vi "Test Person Updates Status on Trigger Broadcast.vi"(8 "error in (no error)":errorcluster, 11 "Person Test In":refnum<class "Person Test.lvclass">) -> (0 "error out":errorcluster, 3 "Person Test Out":refnum<class "Person Test.lvclass">)   [LabVIEW 2020, in "Person Test.lvclass"]
uses:
  Person Test.lvclass
  C:/Program Files (x86)/National Instruments/LabVIEW 2020/vi.lib/Astemes/LUnit/Test Case.lvclass
  Processes/People/Person/Person.lvclass
  C:/Program Files (x86)/National Instruments/LabVIEW 2020/vi.lib/Astemes/Triarc Framework/Process/Process.lvclass
  <vilib>/Astemes/Triarc Framework/Process/Process.lvclass/Process.ctl
  <vilib>/Astemes/LUnit/Test Case.lvclass/Test Case.ctl
  <vilib>/Astemes/Triarc Framework/Process/Private/SubVIs/Wait for finish.vi
  <vilib>/Astemes/Triarc Framework/Process/Private/SubVIs/Set Lifecycle State.vi
  <vilib>/Astemes/Triarc Framework/Process/Protected/Messaging/Send Message.vi
  <vilib>/Astemes/Triarc Framework/Support/Execution timer.vi
  <vilib>/Astemes/LUnit/Core/LUnit Test Case/Private/Append Pass Result.vi
  <vilib>/Astemes/LUnit/Core/LUnit Test Case/Private/Append Fail Result.vi
  d7bc5dd9-32c4-4ae8-b909-84982306f878.vi/9c5d11cd-9439-4240-a1ee-d9baace9c924.vi
  <vilib>/Astemes/Triarc Framework/Process/Private/SubVIs/Handle Debug Data.vi
  <vilib>/Astemes/LUnit/Core/LUnit Test Case/Private/Run In UI.vi
  <vilib>/Astemes/Triarc Framework/Logging/Log Debug.vi
  <vilib>/AdvancedString/1D String Array to Delimited String.vi
  <vilib>/Utility/High Resolution Relative Seconds.vi
  <vilib>/Utility/error.llb/Clear Errors.vi
  <vilib>/Astemes/Triarc Framework/Process/Public/Lifecycle/Get Lifecycle State.vi
  <vilib>/Utility/error.llb/Error Cluster From Error Code.vi
  <vilib>/Astemes/Triarc Framework/Process/Public/Read Name.vi
  <vilib>/Astemes/Triarc Framework/Support/Dequeue Broadcast Message.vi
  <vilib>/Astemes/Triarc Framework/Callback/Callback.lvclass
  <vilib>/Astemes/Triarc Framework/Process/Process.lvclass
  Person Test.lvclass/Person Test.ctl
  <vilib>/Astemes/LUnit/Test Case.lvclass
  <vilib>/Astemes/Triarc Framework/Support/Broadcast Event Dequeuers.lvlib
  1e6db0d7-f4c9-4c1c-b12f-d2d6fb7b9396.vi
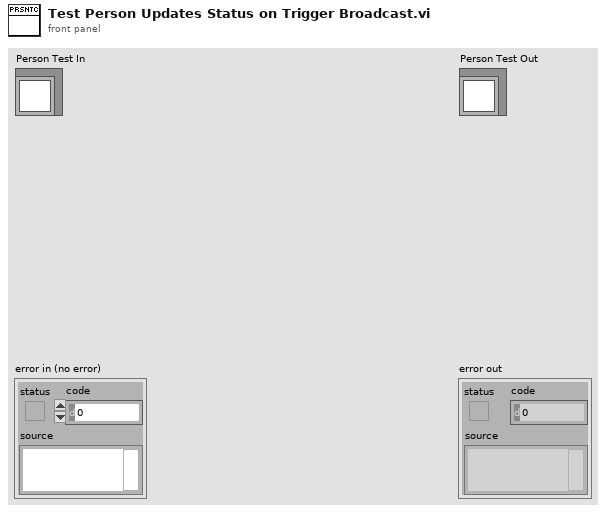
[diagram p1: front panel]
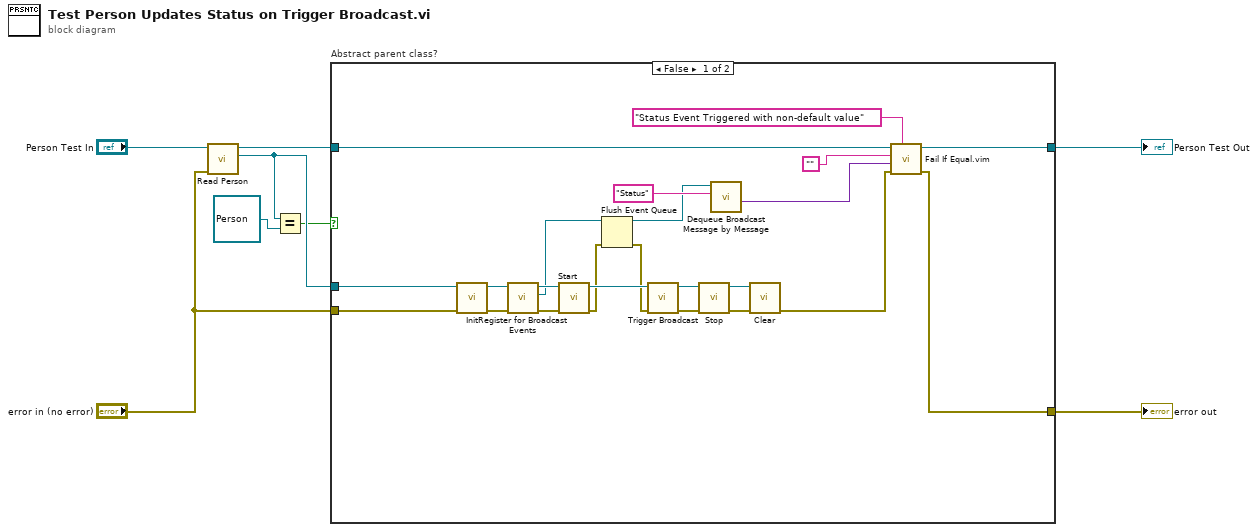
[diagram p0: block diagram]
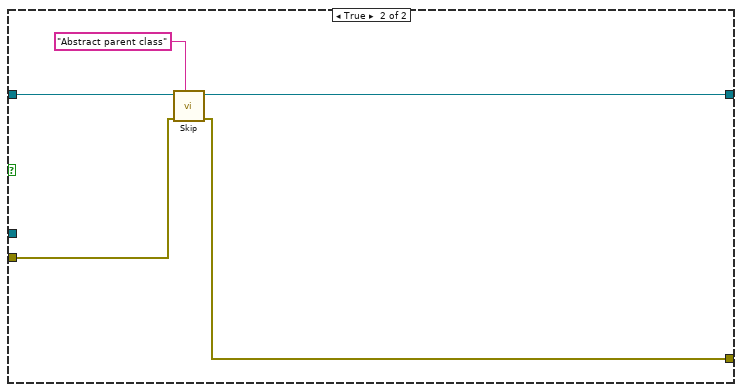
[diagram p2: hidden frame]
diagram:
  n1 = call "Read Person.vi"("error in (no error)"="error in (no error)", "Person Test in"="Person Test In") -> ("Person.lvclass"=w2:refnum<class "Person.lvclass">, "Person Test out"=w7:refnum<class "Person Test.lvclass">)  [unwired: 7 in, 1 out]
  n2 = Equal?(x=w2, y=refnum<class "Person.lvclass"> refnum ("Person.lvclass")) -> (x = y?=w1:bool)
  n3 = case "Abstract parent class?" shown="False" w1 {
    tunnel: w7 -> [w31 w36]
    tunnel: w2 -> [w20 _]
    tunnel: "error in (no error)" -> [w19 w33]
    tunnel: [w16 w35] -> w5
    tunnel: [w9 w32] -> w4
    frame False {
      n4 = call-dynamic "Init.vi"("error in (no error)"=w19, "View In"=w20) -> ("error out"=w29:errorcluster, "View Out"=w30:refnum<class "Person.lvclass">)  [unwired: 8 in]
      n5 = call <vilib>:"Register for Broadcast Events.vi"("error in (no error)"=w29, "Process In"=w30) -> ("error out"=w27:errorcluster, "Event Registration Refnum Out"=w17:refnum<event-registration>, "Process Out"=w28:refnum<class "Person.lvclass">)  [unwired: 7 in]
      n6 = call <vilib>:"Start.vi"("error in (no error)"=w27, "Process In"=w28) -> ("error out"=w25:errorcluster, "Process Out"=w26:refnum<class "Person.lvclass">)  [unwired: 7 in, 1 out]
      n7 = Flush Event Queue(0:w17, 3:w25) -> (8:w11:refnum<event-registration>, 11:w18:errorcluster)  [unwired: 4 in, 1 out]
      n8 = call <vilib>:"Trigger Broadcast.vi"("error in (no error)"=w18, "Process in"=w26) -> ("error out"=w23:errorcluster, "Process out"=w24:refnum<class "Person.lvclass">)  [unwired: 8 in]
      n9 = call <vilib>:"Stop.vi"("error in (no error)"=w23, "Process In"=w24) -> ("error out"=w21:errorcluster, "Process Out"=w22:refnum<class "Person.lvclass">)  [unwired: 7 in, 1 out]
      n10 = call <vilib>:"Dequeue Broadcast Message by Message.vi"("Message"="Status", "Event Registration Refnum"=w11) -> ("Message Data"=w13:variant)  [unwired: 5 in, 4 out]
      n11 = call-dynamic "Clear.vi"("error in (no error)"=w21, "View In"=w22) -> ("error out"=w10:errorcluster)  [unwired: 9 in]
      n12 = call "Fail If Equal.vim"("Description"="Status Event Triggered with non-default value", "error in (no error)"=w10, "Actual"=w13, "Unexpected"="", "LUnit Test Case In"=w31) -> ("error out"=w9:errorcluster, "LUnit Test Case Out"=w16:refnum<class "Person Test.lvclass">)  [unwired: 5 in]
    }
    frame True {
      n13 = call <vilib>:"Skip.vi"("Description"="Abstract parent class", "error in (no error)"=w33, "LUnit Test Case In"=w36) -> ("error out"=w32:errorcluster, "LUnit Test Case Out"=w35:refnum<class "Person Test.lvclass">)  [unwired: 7 in]
    }
  }
  "error out" <- w4
  "Person Test Out" <- w5
